vi "Sample8743UI.vi"() -> ()   [LabVIEW 2009]
uses:
  Global Variables.vi
panel:
  in  "CL Disable":bool
  out "error out":errorcluster
  in  "CL Enable":bool
  out "In Motion":bool
  out "Status:":string
  out "Current Position:":string
  in  "Stop":bool
  in  "Go":bool
  in  "Relative Move:":string
  in  "Selected Motor:":string(combo)
  in  "Selected Controller:":string(combo)
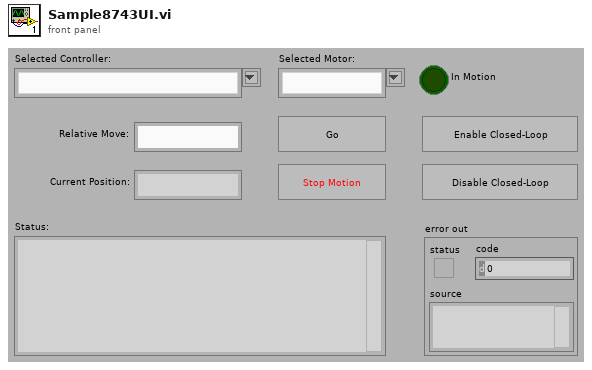
[diagram p1: front panel]
types:
  T1 = cluster{"Selected Controller:":refnum<vi>, "Selected Motor:":refnum<vi>, "Relative Move:":refnum<vi>, "Current Position:":refnum<vi>, "Go":refnum<vi>, "Stop":refnum<vi>, "CL Enable":refnum<vi>, "CL Disable":refnum<vi>}
  T2 = cluster{"DeviceKey":string, "Device Address":i32, "Controller Name":string}[]
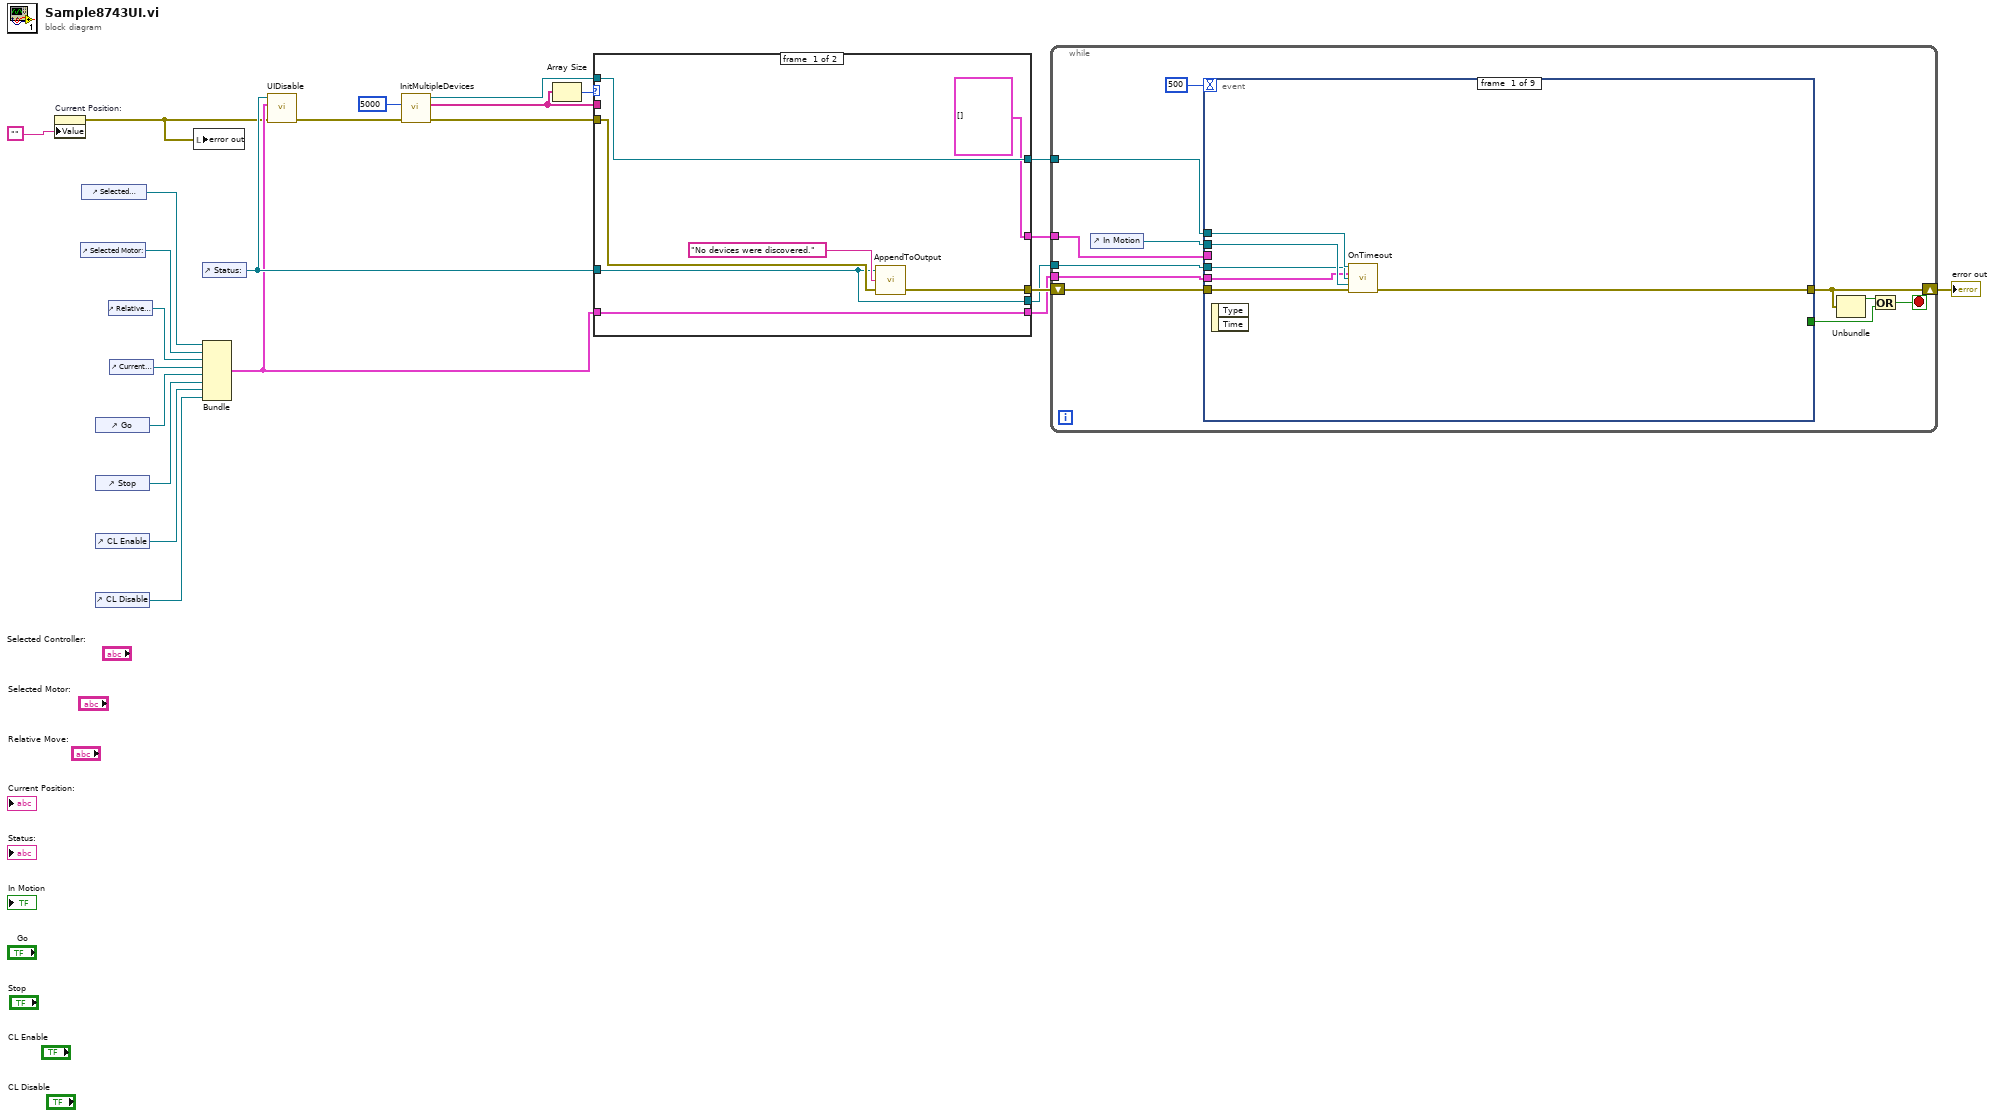
[diagram p0: block diagram]
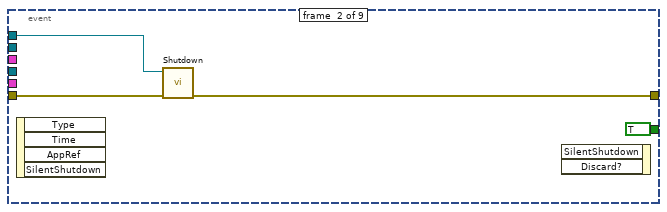
[diagram p2: hidden frame]
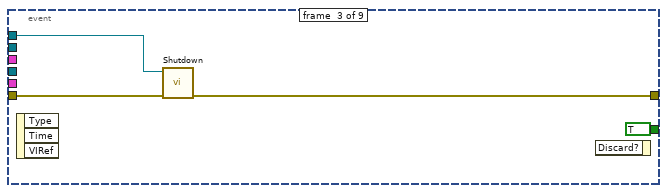
[diagram p3: hidden frame]
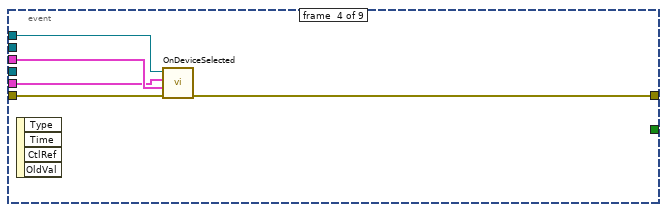
[diagram p4: hidden frame]
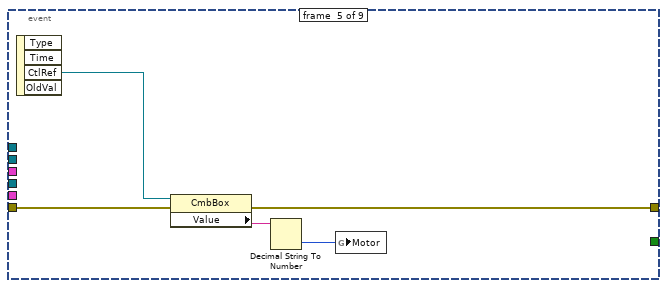
[diagram p5: hidden frame]
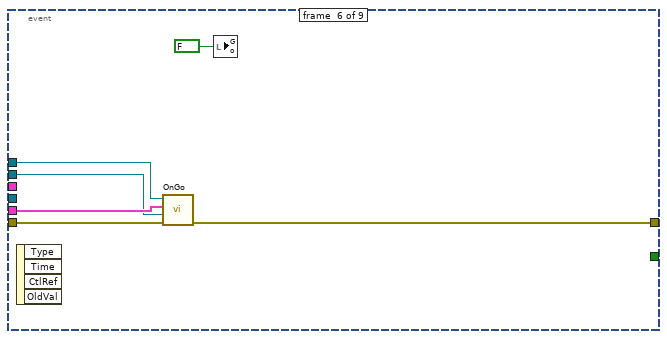
[diagram p6: hidden frame]
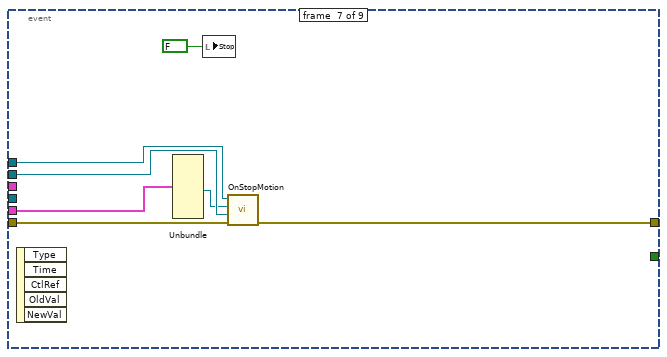
[diagram p7: hidden frame]
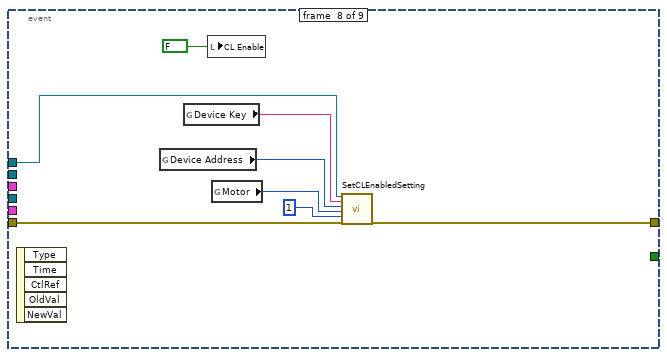
[diagram p8: hidden frame]
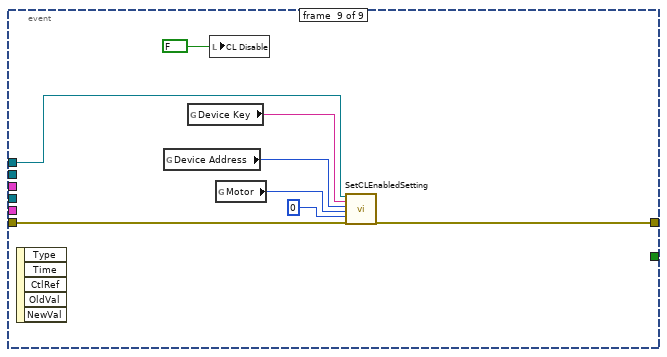
[diagram p9: hidden frame]
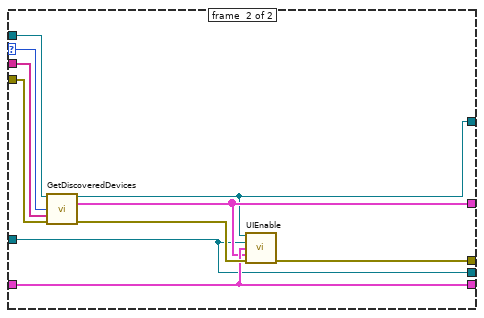
[diagram p10: hidden frame]
diagram:
  n1 = property on="Current Position:" class="Str"("Value"="") -> (error out=w2:errorcluster)  [unwired: 2 in, 1 out]
  n2 = control-ref of="Selected Motor:"() -> (w24:refnum<vi>)
  n3 = control-ref of="Selected Controller:"() -> (w16:refnum<vi>)
  n4 = control-ref of="Go"() -> (w5:refnum<vi>)
  n5 = control-ref of="Stop"() -> (w6:refnum<vi>)
  n6 = control-ref of="CL Enable"() -> (w7:refnum<vi>)
  n7 = control-ref of="CL Disable"() -> (w1:refnum<vi>)
  n8 = control-ref of="Relative Move:"() -> (w23:refnum<vi>)
  n9 = control-ref of="Current Position:"() -> (w4:refnum<vi>)
  n10 = local write "error out"(w2) -> ()
  n11 = control-ref of="Status:"() -> (w15:refnum<vi>)
  n12 = Bundle("Selected Controller:"=w16, "Selected Motor:"=w24, "Relative Move:"=w23, "Current Position:"=w4, "Go"=w5, "Stop"=w6, "CL Enable"=w7, "CL Disable"=w1) -> (w11:T1)  [unwired: 1 in]
  n13 = call "UIDisable.vi"("error in (no error)"=w2, "UI"=w11, "Status:"=w15) -> ("error out"=w22:errorcluster)  [unwired: 8 in]
  n14 = call "InitMultipleDevices.vi"("error in (no error)"=w22, "msecDelayForDiscovery"=5000) -> ("error out"=w19:errorcluster, "DeviceKey List Out"=w17:string[], "CmdLib Out"=w18:refnum<k24>)  [unwired: 3 in]
  n15 = Array Size(array=w17) -> (size(s)=w20:i32)
  n16 = case shown="1, Default" w20 {
    selector: w20 -> [_ w37]
    tunnel: w15 -> [w25 w32]
    tunnel: w19 -> [w30 w40]
    tunnel: w18 -> [w28 w41]
    tunnel: w17 -> [_ w39]
    tunnel: [w29 w36] -> w14
    tunnel: [w28 w33] -> w13
    tunnel: w11 -> [w27 w35]
    tunnel: [w27 w35] -> w9
    tunnel: [T2 [] ("Device Array") w34] -> w8
    tunnel: [w25 w32] -> w3
    frame #0 {
      n17 = call "AppendToOutput.vi"("error in"=w30, "Input String"="No devices were discovered.", "Output Refnum In"=w25) -> ("error out"=w29:errorcluster)  [unwired: 1 in, 1 out]
    }
    frame #1 {
      n18 = call "GetDiscoveredDevices.vi"("CmdLib In"=w41, "Master Count"=w37, "DeviceKey List"=w39, "error in"=w40) -> ("CmdLib Out"=w33:refnum<k24>, "Device Array"=w34:T2, "error out"=w38:errorcluster)  [unwired: 9 in]
      n19 = call "UIEnable.vi"("CmdLib In"=w33, "Status:"=w32, "UI"=w35, "Device Array"=w34, "error in"=w38) -> ("error out"=w36:errorcluster)  [unwired: 10 in]
    }
  }
  n20 = while {
    tunnel: w13 -> [w51]
    tunnel: w9 -> [w50]
    tunnel: w8 -> [w49]
    shift-right: [w46] -> w10
    shift-left: w14 -> [w52]
    tunnel: w3 -> [w47]
    stop <- w45 stop-if-true
    n21 = control-ref of="In Motion"() -> (w42:refnum<vi>)
    n22 = event shown="[8] \"CL Disable\": Value Change" {
      selector: _ -> [_ _ _ _ _ _ _ _ _]
      dyn-events: _ -> [_ _ _ _ _ _ _ _ _]
      timeout: 500 -> [_ _ _ _ _ _ _ _ _]
      tunnel: w52 -> [w58 w62 w65 w71 w74 w82 w88 w91 w99]
      tunnel: w51 -> [w55 w61 w66 w67 _ w80 w87 w90 w101]
      tunnel: [_ TRUE TRUE _ _ _ _ _ _] -> w43
      tunnel: [w57 w59 w63 w70 w73 w77 w85 w92 w100] -> w46
      tunnel: w50 -> [w53 _ _ w68 _ w81 w84 _ _]
      tunnel: w49 -> [_ _ _ w69 _ _ _ _ _]
      tunnel: w47 -> [w54 _ _ _ _ _ _ _ _]
      tunnel: w42 -> [w56 _ _ _ _ w79 w89 _ _]
      event #0 {
        n23 = event-data() -> ()  [unwired: 1 in, 2 out]
        n24 = call "OnTimeout.vi"("CmdLib In"=w55, "UI"=w53, "Status:"=w54, "In Motion"=w56, "error in"=w58) -> ("error out"=w57:errorcluster)  [unwired: 10 in]
      }
      event #1 {
        n25 = event-data() -> ()  [unwired: 1 in, 4 out]
        n26 = call "Shutdown.vi"("error in (no error)"=w62, "CmdLib In"=w61) -> ("error out"=w59:errorcluster)  [unwired: 4 in, 1 out]
        n27 = event-data() -> ()  [unwired: 3 in, 1 out]
      }
      event #2 {
        n28 = event-data() -> ()  [unwired: 1 in, 3 out]
        n29 = call "Shutdown.vi"("error in (no error)"=w65, "CmdLib In"=w66) -> ("error out"=w63:errorcluster)  [unwired: 4 in, 1 out]
        n30 = event-data() -> ()  [unwired: 2 in, 1 out]
      }
      event #3 {
        n31 = event-data() -> ()  [unwired: 1 in, 4 out]
        n32 = call "OnDeviceSelected.vi"("error in"=w71, "Device Array"=w69, "UI"=w68, "CmdLib In"=w67) -> ("error out"=w70:errorcluster)  [unwired: 7 in]
      }
      event #4 {
        n33 = event-data() -> ("CtlRef"=w72:refnum<vi>)  [unwired: 1 in, 3 out]
        n34 = property class="CmbBox"(reference=w72, error in=w74) -> (error out=w73:errorcluster, "Value"=w76:string)  [unwired: 1 out]
        n35 = Decimal String To Number(string=w76) -> (number=w75:i32)  [unwired: 2 in, 1 out]
        n36 = global write "Global Variables.vi" "Motor"(w75) -> ()
      }
      event #5 {
        n37 = event-data() -> ()  [unwired: 1 in, 4 out]
        n38 = call "OnGo.vi"("error in"=w82, "In Motion"=w79, "UI"=w81, "CmdLib Out"=w80) -> ("error out"=w77:errorcluster)  [unwired: 7 in]
        n39 = local write "Go"(FALSE ("Go")) -> ()
      }
      event #6 {
        n40 = event-data() -> ()  [unwired: 1 in, 5 out]
        n41 = Unbundle(w84) -> ("Go"=w83:refnum<vi>)  [unwired: 7 out]
        n42 = local write "Stop"(FALSE ("Stop")) -> ()
        n43 = call "OnStopMotion.vi"("error in"=w88, "In Motion"=w89, "Go"=w83, "CmdLib In"=w87) -> ("error out"=w85:errorcluster)  [unwired: 7 in]
      }
      event #7 {
        n44 = event-data() -> ()  [unwired: 1 in, 5 out]
        n45 = global read "Global Variables.vi" "Device Address"() -> (w96:i32)
        n46 = global read "Global Variables.vi" "Device Key"() -> (w95:string)
        n47 = local write "CL Enable"(FALSE ("CL Enable")) -> ()
        n48 = global read "Global Variables.vi" "Motor"() -> (w94:i32)
        n49 = call "SetCLEnabledSetting.vi"("CmdLib In"=w90, "DeviceKey In"=w95, "Device Address In"=w96, "Motor"=w94, "Setting"=1 ("t"), "error in (no error)"=w91) -> ("error out"=w92:errorcluster)  [unwired: 10 in, 3 out]
      }
      event #8 {
        n50 = event-data() -> ()  [unwired: 1 in, 5 out]
        n51 = global read "Global Variables.vi" "Device Address"() -> (w102:i32)
        n52 = global read "Global Variables.vi" "Device Key"() -> (w103:string)
        n53 = local write "CL Disable"(FALSE ("CL Disable")) -> ()
        n54 = global read "Global Variables.vi" "Motor"() -> (w104:i32)
        n55 = call "SetCLEnabledSetting.vi"("CmdLib In"=w101, "DeviceKey In"=w103, "Device Address In"=w102, "Motor"=w104, "Setting"=0 ("t"), "error in (no error)"=w99) -> ("error out"=w100:errorcluster)  [unwired: 10 in, 3 out]
      }
    }
    n56 = Unbundle(w46) -> ("status"=w44:bool)  [unwired: 2 out]
    n57 = Or(x=w44, y=w43) -> (x .or. y?=w45:bool)
  }
  "error out" <- w10
